vi "HC MFR sw 2.vi"(8 "Increment":dbl, 9 "HC Conc %":dbl, 10 "C_HC":dbl, 11 "Flow rate":dbl) -> (3 "HC MFR":dbl)   [LabVIEW 2014]
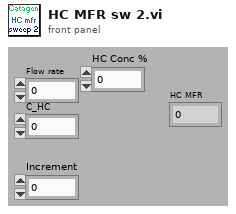
[diagram p1: front panel]
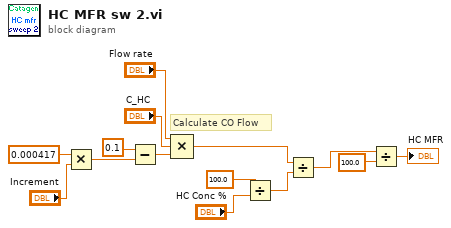
[diagram p0: block diagram]
diagram:
  # "Calculate CO Flow"
  n1 = Multiply(x=0.000417, y="Increment") -> (x*y=w9:dbl)
  n2 = Subtract(x=0.1, y=w9) -> (x-y=w6:dbl)
  n3 = Compound Arithmetic op=MULTIPLY("Flow rate", "C_HC", w6) -> (w2:dbl)
  n4 = Divide(x=100.0, y="HC Conc %") -> (x/y=w3:dbl)
  n5 = Divide(x=w2, y=w3) -> (x/y=w1:dbl)
  n6 = Divide(x=w1, y=100.0) -> (x/y=→"HC MFR":dbl)
